vi "GetInstrumentFolders.vi"() -> (3 "folder names":string[](array[string]))   [LabVIEW 2022 SP3]
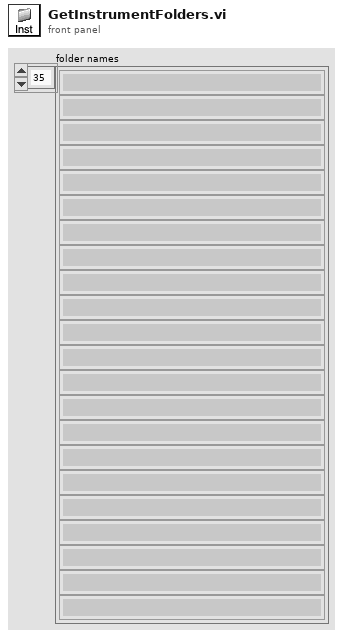
[diagram p1: front panel]
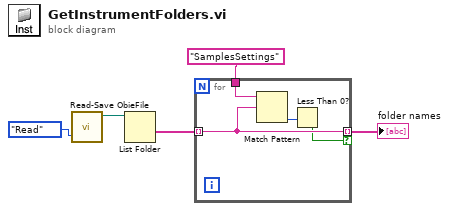
[diagram p0: block diagram]
diagram:
  n1 = call "Read-Save ObieFile.vi"("Task"=enum16{"Save", "Read"}."Read") -> ("DataPath Out"=w4:path)  [unwired: 8 in, 2 out]
  n2 = List Folder(path=w4) -> (folder names=w3:string[])  [unwired: 3 in, 3 out]
  n3 = for {
    tunnel: [w8] -> w2 mode=indexing if=w6
    tunnel: w3 -> [w8] mode=indexing
    tunnel: "SamplesSettings" -> [w9]
    n4 = Match Pattern(string=w9, regular expression=w8) -> (offset past match=w7:i32)  [unwired: 1 in, 3 out]
    n5 = Less Than 0?(x=w7) -> (x < 0?=w6:bool)
  }
  "folder names" <- w2
